vi "PH_Synchrolock_Watch.constructor.vi"(0 "name":string, 2 "data in":string, 5 "error in(no error)":errorcluster) -> (14 "i ref out":refnum<vi>, 16 "data out":string, 19 "error out":errorcluster)   [LabVIEW 2014, in "PH_Synchrolock_Watch.lvlib"]
doc: "This is the constructor of a class.\n\nLicense Agreement for this software:\n\nCopyright (C)\nGesellschaft für Schwerionenforschung, GSI\nPlanckstr. 1\n64291 Darmstadt\nGermany\n\nContact: D.Beck@gsi.de \n\nThis program is free software; you can redistribute it and/or modify it under the terms of the \nGNU General Public License as published by the Free Software Foundation; either version 2 of \nthe license, or (at your option) any later version.\n\nThis program is distributed in the hope that it will be useful, but WITHOUT ANY WARRANTY; \nwithout even the implied warranty of MERCHANTABILITY or FITNESS FOR A PARTICULAR PURPOSE. See the GNU General License for more details (http://www.gnu.org).\n\nGesellschaft für Schwerionenforschung, GSI\nPlanckstr. 1, 64291 Darmstadt, Germany\nFor all questions and ideas contact: M.Richter@gsi.de, H.Brand@gsi.de or D.Beck@gsi.de.\nLast update: 16-JUN-2004"
uses:
  PH_Synchrolock_Watch.lvlib
  PH_Synchrolock_Watch.i attribute.ctl
  CS_Core/CSSystem/CSSystemLib/CSSystemLib.lvlib
  PH_Devices/PH_TKTDS-30xx/PH_TKTDS-30xx.lvlib
  CS_Core/CSObj/CSObj.lvlib
  PH_Basics/PH_Class/PH_Class.lvlib
  PH_Basics/PH_StatusHandler/PH_StatusHandler.lvlib
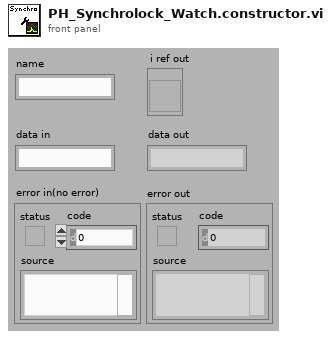
[diagram p1: front panel]
types:
  T1 = typedef "PH_Synchrolock_Watch.lvlib/PH_Synchrolock_Watch.i attribute.ctl" = cluster{"GUI Refs":cluster{"Mean Phase Graph":refnum<vi>, "RF Amplitude Graph":refnum<vi>, "Mira Amplitude Graph":refnum<vi>, "MIRA State":refnum<vi>, "Mean Phase":refnum<vi>, "RF Amplitude":refnum<vi>, "Mira Amplitude":refnum<vi>, "Mean Phase in range?":refnum<vi>, "RF Amplitude above limit?":refnum<vi>, "Mira Amplitude in range?":refnum<vi>, "Mean phase upper limit":refnum<vi>, "Mean phase lower limit":refnum<vi>, "RF Amplitude lower limit":refnum<vi>, "Mira Amplitude lower limit":refnum<vi>, "Mira Amplitude upper limit":refnum<vi>, "Mira scope":refnum<vi>, "Reset Mira warning":refnum<vi>}, "Status":cluster{"Reset Warning":bool}, "Mean Phase":cluster{"Current Value":dbl, "Upper Limit":dbl, "Lower Limit":dbl, "Data":cluster{dbl[], dbl[]}}, "RF":cluster{"Current Value":dbl, "Lower Limit":dbl, "Data":cluster{dbl[], dbl[]}}, "MIRA":cluster{"Current Value":dbl, "Upper Limit":dbl, "Lower Limit":dbl, "Data":cluster{dbl[], dbl[]}}}
  T2 = enum16{"SetAttribute", "GetAttribute", "CreateAttribute", "DestroyAttribute", "DestroyAllAtributes"}
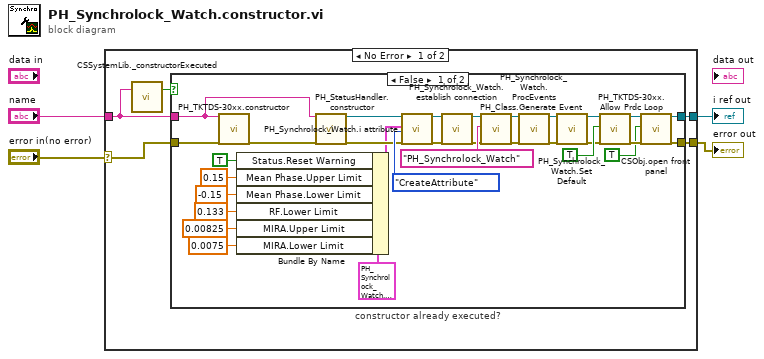
[diagram p0: block diagram]
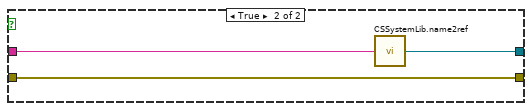
[diagram p2: hidden frame]
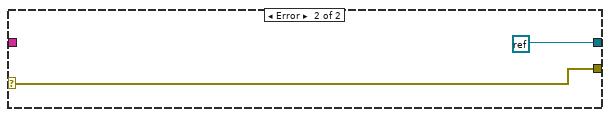
[diagram p3: hidden frame]
diagram:
  n1 = case shown="No Error" "error in(no error)" {
    selector: "error in(no error)" -> [w7 w44]
    tunnel: "name" -> [w6 _]
    tunnel: [w9 refnum<k0> refnum] -> w3
    tunnel: [w8 w44] -> w2
    frame No Error {
      n2 = call "CSSystemLib._constructorExecuted.vi"("name"=w6) -> ("constructor executed?"=w5:bool)  [unwired: 18 in]
      n3 = case "constructor already executed?" shown="False" w5 {
        tunnel: [w37 w42] -> w9
        tunnel: [w35 w41] -> w8
        tunnel: w7 -> [w11 w41]
        tunnel: w6 -> [w10 w43]
        frame False {
          n4 = call "PH_TKTDS-30xx.constructor.vi"("name"=w10, "error in(no error)"=w11) -> ("error out"=w27:errorcluster)  [unwired: 15 in, 2 out]
          n5 = Bundle By Name(cluster=T1 {"GUI Refs"={"Mean Phase Graph"=refnum, "RF Amplitude Graph"=refnum, "Mira Amplitude Graph"=refnum, "MIRA State"=refnum, "Mean Phase"=refnum, "RF Amplitude"=refnum, "Mira Amplitude"=refnum, "Mean Phase in range?"=refnum, "RF Amplitude above limit?"=refnum, "Mira Amplitude in range?"=refnum, "Mean phase upper limit"=refnum, "Mean phase lower limit"=refnum, "RF Amplitude lower limit"=refnum, "Mira Amplitude lower limit"=refnum, "Mira Amplitude upper limit"=refnum, "Mira scope"=refnum, "Reset Mira warning"=refnum}, "Status"={"Reset Warning"=FALSE}, "Mean Phase"={"Current Value"=0.0, "Upper Limit"=0.0, "Lower Limit"=0.0, "Data"={[], []}}, "RF"={"Current Value"=0.0, "Lower Limit"=0.0, "Data"={[], []}}, "MIRA"={"Current Value"=0.0, "Upper Limit"=0.0, "Lower Limit"=0.0, "Data"={[], []}}} ("i attribute"), "Status.Reset Warning"=TRUE, "Mean Phase.Upper Limit"=0.15, "Mean Phase.Lower Limit"=-0.15, "RF.Lower Limit"=0.133, "MIRA.Upper Limit"=0.00825, "MIRA.Lower Limit"=0.0075) -> (w28:T1)
          n6 = call "PH_StatusHandler.constructor.vi"("name"=w10, "error in(no error)"=w27) -> ("i ref out"=w30:refnum<vi>, "error out"=w29:errorcluster)  [unwired: 15 in, 1 out]
          n7 = call "PH_Synchrolock_Watch.i attribute.vi"("VI Refnum"=w30, "CLASS.i attribute"=w28, "Action"=T2."CreateAttribute", "error in (no error)"=w29) -> ("VI Refnum out"=w26:refnum<vi>, "error out"=w25:errorcluster)  [unwired: 13 in, 1 out]
          n8 = call "PH_Synchrolock_Watch.establish connection.vi"("i ref in"=w26, "error in"=w25) -> ("i ref out"=w13:refnum<vi>, "error out"=w12:errorcluster)  [unwired: 16 in]
          n9 = call "PH_Class.Generate Event.vi"("i ref in"=w13, "Class"="PH_Synchrolock_Watch", "error in (no error)"=w12) -> ("i ref out"=w24:refnum<vi>, "error out"=w23:errorcluster)  [unwired: 15 in]
          n10 = call "PH_Synchrolock_Watch.ProcEvents.vi"("i ref in"=w24, "error in"=w23) -> ("i ref out"=w38:refnum<vi>, "error out"=w39:errorcluster)  [unwired: 16 in]
          n11 = call "PH_Synchrolock_Watch.Set Default.vi"("i ref in"=w38, "error in"=w39) -> ("i ref out"=w21:refnum<vi>, "error out"=w20:errorcluster)  [unwired: 16 in]
          n12 = call "PH_TKTDS-30xx.Allow Prdc Loop.vi"("i ref in"=w21, "Allow Prdc Loop?"=TRUE ("Contructor finished"), "error in"=w20) -> ("i ref out"=w36:refnum<vi>, "error out"=w34:errorcluster)  [unwired: 15 in]
          n13 = call "CSObj.open front panel.vi"("i ref in"=w36, "frontPanelOpen"=TRUE, "error in (no error)"=w34) -> ("i ref out"=w37:refnum<vi>, "error out"=w35:errorcluster)  [unwired: 15 in]
        }
        frame True {
          n14 = call "CSSystemLib.name2ref.vi"("name"=w43) -> ("obj refnum"=w42:refnum<vi>)
        }
      }
    }
    frame Error {
    }
  }
  "i ref out" <- w3
  "error out" <- w2
